vi "WS - Wait for motion stop.vi"(4 "Delay":dbl format="%.2f", 6 "error in":errorcluster, 8 "Axis  #":i8=1 min=1 max=6 step=1, 9 "Address / Port":i16=1 min=1 max=31 step=1) -> (0 "error out":errorcluster, 2 "Axis  # dup":i8=1 min=1 max=6 step=1, 3 "Address / Port dup":i16=1 min=1 max=31 step=1)   [LabVIEW 2014]
doc: "Wait for the end of the movement of the motor set on \"Axis#\".\nIt is possible to set a \"Delay\" to wait after the movement is over."
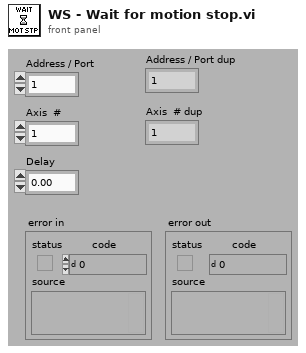
[diagram p1: front panel]
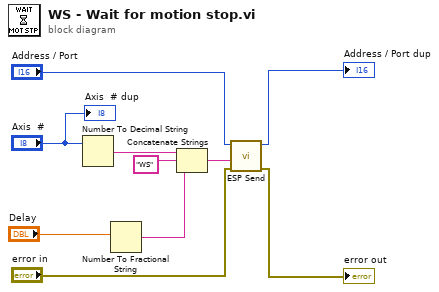
[diagram p0: block diagram]
diagram:
  n1 = Number To Decimal String(number="Axis  #") -> (decimal integer string=w9:string)  [unwired: 1 in]
  n2 = Number To Fractional String(number="Delay") -> (F-format string=w3:string)  [unwired: 3 in]
  n3 = Concatenate Strings(w9, "WS" ("Substring"), w3) -> (w7:string)
  n4 = call "ESP Send.vi"("error in"="error in", "Command String"=w7, "Address / Port"="Address / Port") -> ("error out"=→"error out":errorcluster, "Address / Port dup"=→"Address / Port dup":i16)  [unwired: 3 in]
  "Axis  # dup" <- "Axis  #"
